vi "储液罐状态监控前面板.vi"() -> ()   [LabVIEW 2010]
panel:
  out "波形图表":dbl(graph)
  out "液位超标":bool
  in  "停止":bool
  in  "手动    自动":bool
  in  "设定高度(m)":dbl(slide)=3.4545454545454546 scale=0.0..10.0
  out "温度(℃)":dbl(slide)=53.271 scale=0.0..100.0
  out "实际液位(m)":dbl(slide)=3.31 scale=0.0..10.0
  in  "调节步长":dbl(knob)=5.0 min=5.0 max=20.0 step=1.0 scale=0.0..10.0 scale format="%#.0f"
  out "压力(MPa)":cluster{dbl, dbl}(knob)={2.06, 1.6} scale=0.0..5.0 scale format="%#_2f"
  out "液位超标":bool
  # "储 液 罐 状 态 监 测"
  # "进口压力"
  # "出口压力"
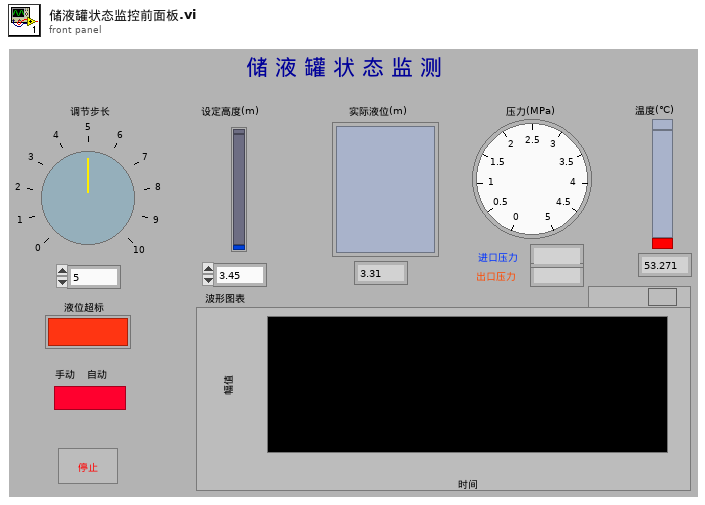
[diagram p1: front panel]
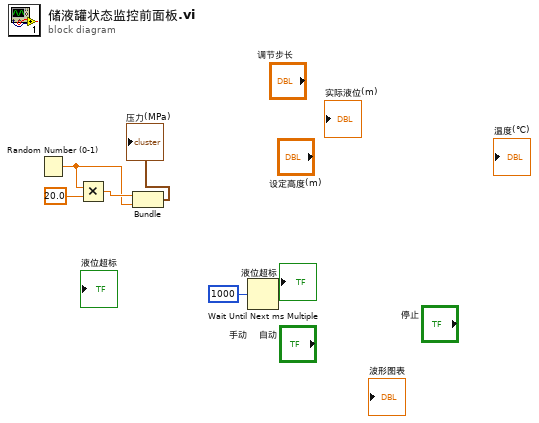
[diagram p0: block diagram]
diagram:
  n1 = Random Number (0-1)() -> (number: 0 to 1=w3:dbl)
  n2 = Multiply(x=w3, y=20.0) -> (x*y=w4:dbl)
  n3 = Bundle(w4, "number: 0 to 1"=w3) -> (→"压力(MPa)":cluster{dbl, "number: 0 to 1":dbl})  [unwired: 1 in]
  n4 = Wait Until Next ms Multiple(millisecond multiple=u32 1000 ("毫秒倍数")) -> ()  [unwired: 1 out]
